vi "Reset Request.vi"(8 "error in (no error)":errorcluster, 11 "FHPP in":refnum<class "FHPP.lvclass">) -> (0 "error out":errorcluster)   [LabVIEW 2022 SP3, in "FHPP.lvclass"]
uses:
  FHPP.lvclass
  FHPP.lvclass/FHPP.ctl
  TypeDefs/ReqID.ctl
  TypeDefs/FCT Request.ctl
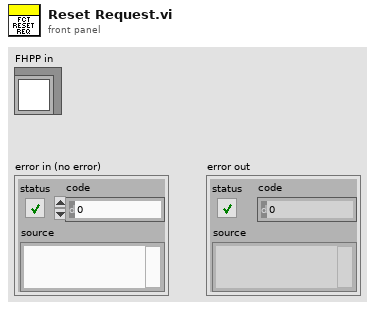
[diagram p1: front panel]
types:
  T1 = typedef "FHPP.lvclass/FCT Request.ctl" = cluster{"Request":T2, "PNU":u16, "Subindex":u16, "Data":u32}
  T2 = typedef "FHPP.lvclass/ReqID.ctl" = u8
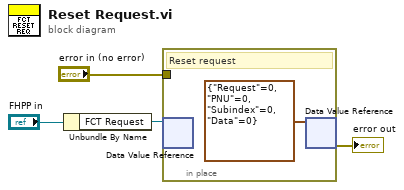
[diagram p0: block diagram]
diagram:
  n1 = Unbundle By Name("FHPP in") -> ("FCT Request"=w3:refnum<data-value>)
  n2 = in-place {
    in-place-border: "error in (no error)" -> [_]
    # "Reset request"
    n3 = in-place-dvr #1(w3) -> ()  [unwired: 2 out]
    n4 = in-place-dvr #1(T1 {"Request"=0, "PNU"=0, "Subindex"=0, "Data"=0} ("data value")) -> (→"error out":errorcluster)  [unwired: 1 out]
  }
